vi "Simulation_WorkingArea.vi"(10 "L 2":dbl(slide)=77.0 scale=0.0..200.0, 11 "L 1":dbl(slide)=77.0 scale=0.0..200.0) -> (1 "2D Picture 2":picture, 2 "XY Graph 2":cluster{"X":dbl, "Y":dbl}[](graph), 3 "Array":cluster{dbl, dbl}[](array[cluster]))   [LabVIEW 2024]
panel:
  out "2D Picture 3":picture
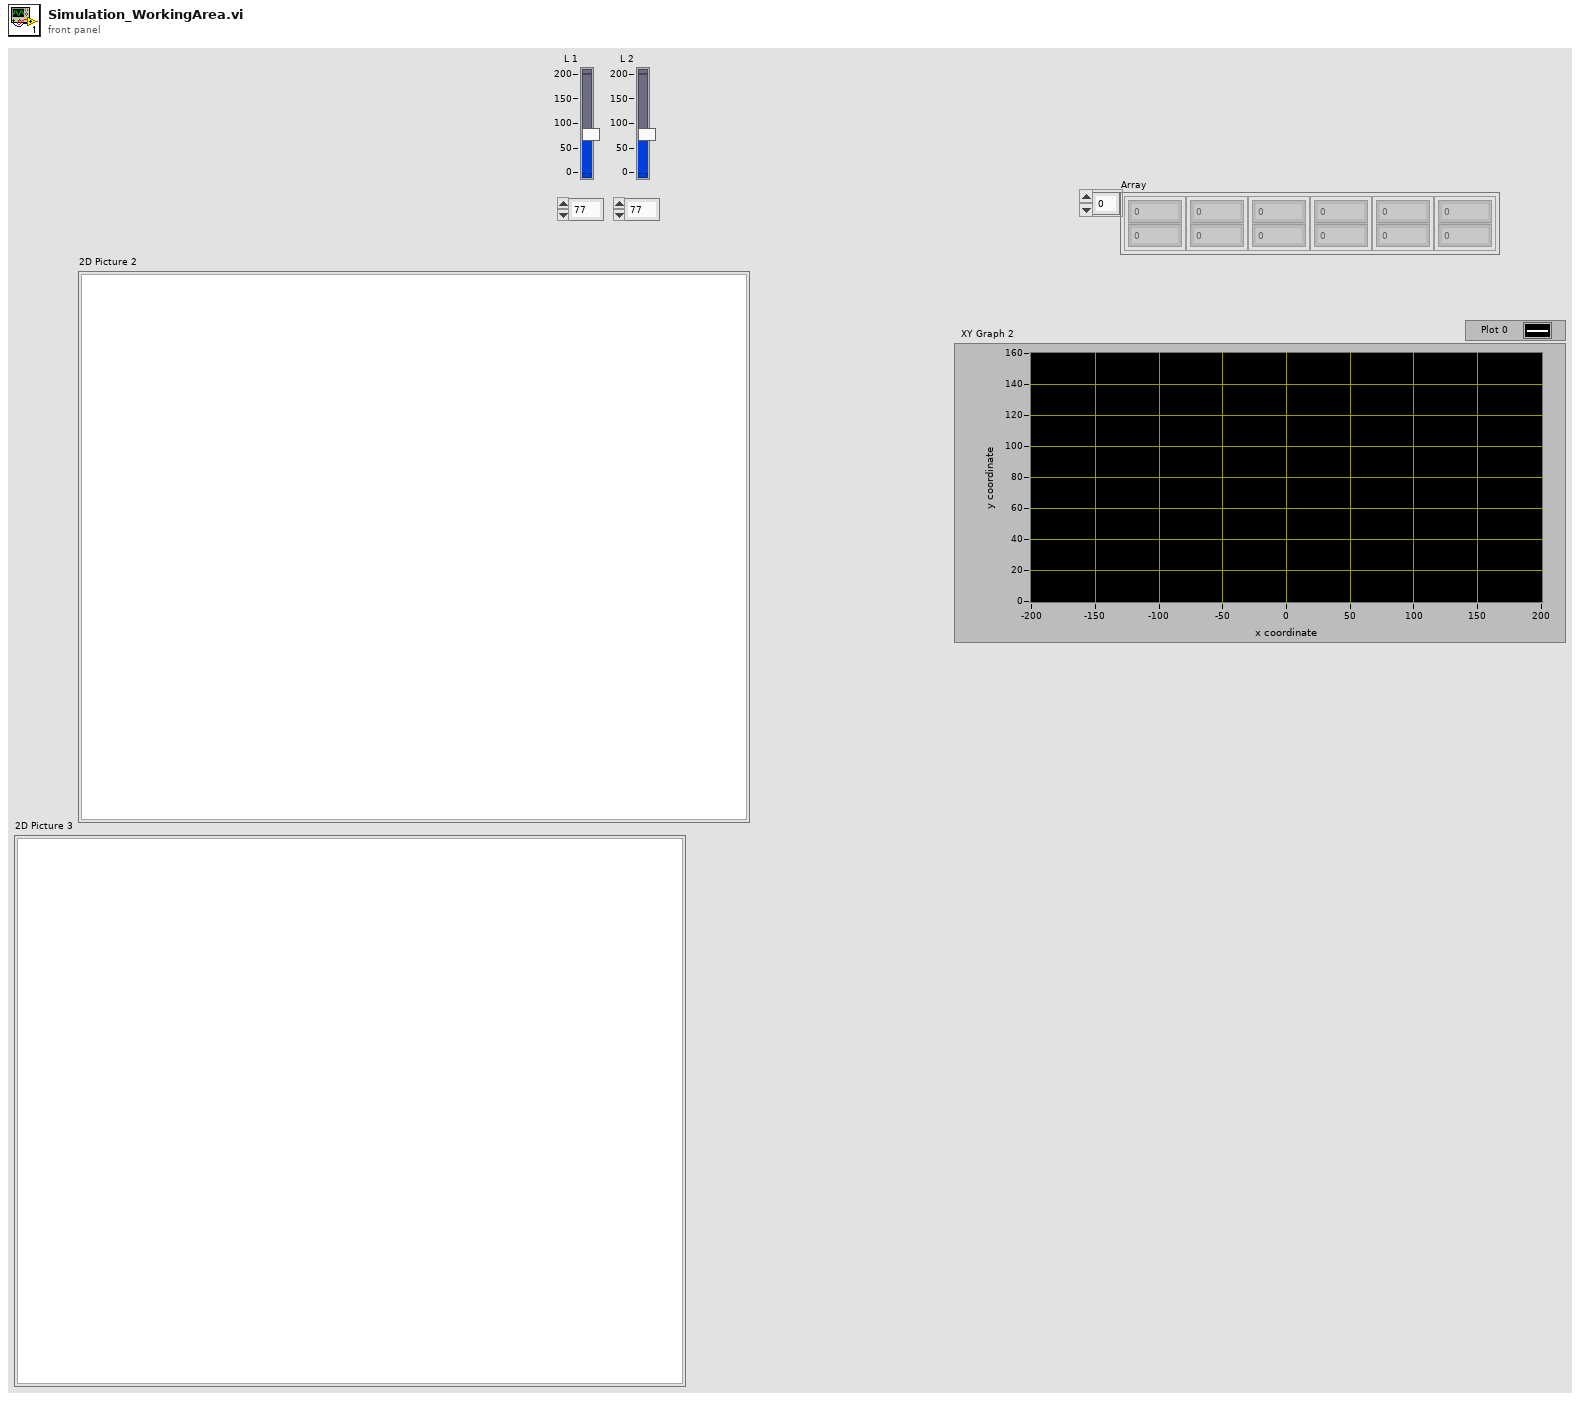
[diagram p1: front panel]
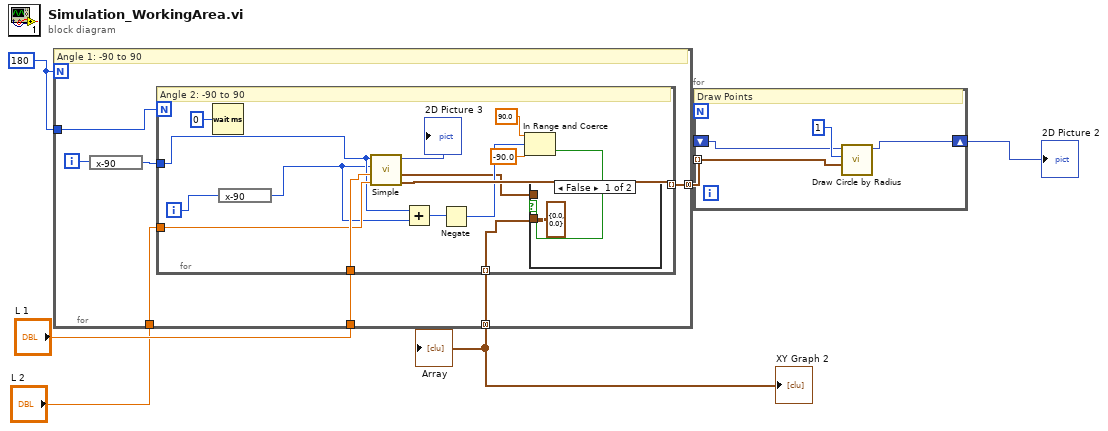
[diagram p0: block diagram]
diagram:
  w6 = 180
  n1 = for {
    N: w6 -> [_]
    tunnel: w6 -> [w13]
    tunnel: [w11] -> w5 mode=concatenating
    tunnel: [w8] -> w1 mode=concatenating
    tunnel: "L 1" -> [w10]
    tunnel: "L 2" -> [w9]
    i -> [w7]
    # "Angle 1: -90 to 90"
    n2 = expression code="x-90"(w7) -> (w12:i32)
    n3 = for {
      N: w13 -> [_]
      tunnel: w12 -> [w15]
      tunnel: [w27] -> w11 mode=indexing
      tunnel: [w17] -> w8 mode=indexing
      tunnel: w10 -> [w24]
      tunnel: w9 -> [w23]
      i -> [w28]
      # "Angle 2: -90 to 90"
      n4 = Wait (ms)(milliseconds to wait=u32 0) -> ()  [unwired: 1 out]
      n5 = expression code="x-90"(w28) -> (w14:i32)
      n6 = call "Simple.vi"("L 2"=w23, "L 1"=w24, "Angle 2"=w14, "Angle1"=w15) -> ("Final 2D Pos"=w27:cluster{dbl, dbl}, "end effector"=w16:cluster{dbl, dbl}, "2D Picture"=→"2D Picture 3":picture)  [unwired: 5 in]
      n7 = Add(x=w15, y=w14) -> (x+y=w22:i32)
      n8 = Negate(x=w22) -> (-x=w19:i32)
      n9 = In Range and Coerce(upper limit=90.0, x=w19, lower limit=-90.0) -> (In Range?=w18:bool)  [unwired: 1 out]
      n10 = case shown="False" w18 {
        tunnel: [cluster{dbl, dbl} {0.0, 0.0} ("end effector") w30] -> w17
        tunnel: w16 -> [_ w30]
        frame False {
        }
        frame True {
        }
      }
    }
  }
  "XY Graph 2" <- w1
  "Array" <- w1
  n11 = for {
    tunnel: w5 -> [w31] mode=indexing
    shift-right: [w33] -> w4
    shift-left: _ -> [w32]
    # "Draw Points"
    n12 = call <vilib>:"Draw Circle by Radius.vi"("pixel center"=w31, "radius"=i16 1, "picture"=w32) -> ("new picture"=w33:picture)  [unwired: 8 in]
  }
  "2D Picture 2" <- w4
